vi "Split_Ch_name.vi"(0 "Ch name":string) -> (1 "Top level":string, 2 "Middle":string, 3 "Low level":string)   [LabVIEW 2010]
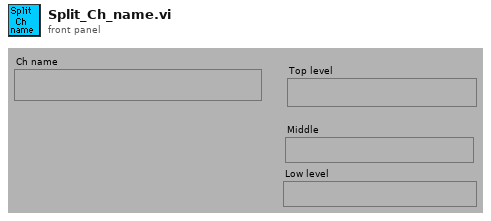
[diagram p1: front panel]
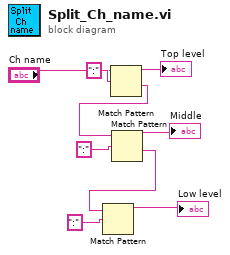
[diagram p0: block diagram]
diagram:
  n1 = Match Pattern(string="Ch name", regular expression=":") -> (before substring=→"Top level":string, after substring=w8:string)  [unwired: 3 out]
  n2 = Match Pattern(string=w8, regular expression=":") -> (before substring=→"Middle":string, after substring=w2:string)  [unwired: 3 out]
  n3 = Match Pattern(string=w2, regular expression=":") -> (before substring=→"Low level":string)  [unwired: 4 out]
